vi "Wait For Goal.vi"(6 "Side":T1, 7 "wait time":dbl, 8 "error in":errorcluster, 10 "Goal":dbl[](array[numeric])) -> (0 "error out":errorcluster, 3 "Aborted":bool)   [LabVIEW 2013]
uses:
  ROS/Code/SubVIs/BaxterSide.ctl
  Arm Globals.vi
  ROS/Code/Console/Servers/ServerSubs/(nist) Arm Globals.vi
panel:
  in  "Label":string
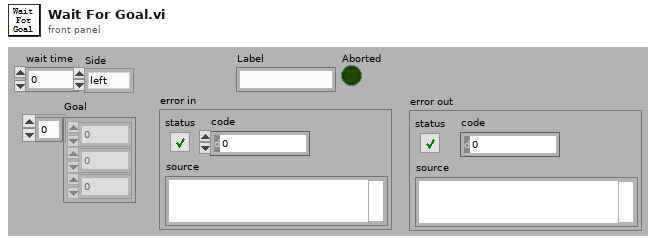
[diagram p1: front panel]
types:
  T1 = typedef "BaxterSide.ctl" = enum16{"left", "right"}
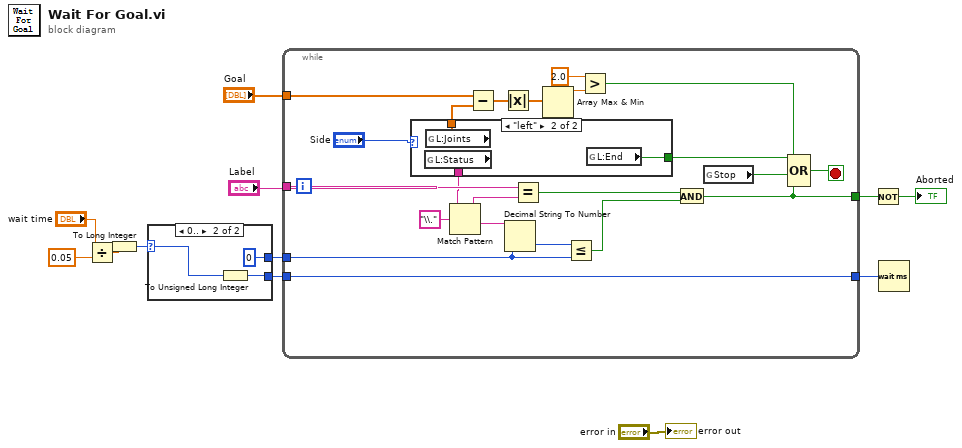
[diagram p0: block diagram]
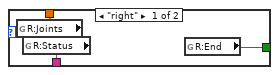
[diagram p2: hidden frame]
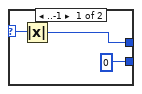
[diagram p3: hidden frame]
diagram:
  n1 = Divide(x="wait time", y=0.05) -> (x/y=w7:dbl)
  n2 = To Long Integer(number=w7) -> (32bit integer=w6:i32)
  n3 = case shown="0.." w6 {
    selector: w6 -> [w15 w17]
    tunnel: [w13 0] -> w11
    tunnel: [u32 0 w18] -> w10
    frame ..-1 {
      n4 = Absolute Value(x=w15) -> (abs(x)=w13:i32)
    }
    frame 0.. {
      n5 = To Unsigned Long Integer(number=w17) -> (unsigned 32bit integer=w18:u32)
    }
  }
  n6 = while {
    tunnel: "Label" -> [w40]
    tunnel: [w28] -> w4
    tunnel: w11 -> [w31]
    tunnel: w10 -> [w30]
    tunnel: [w30] -> w2
    tunnel: "Goal" -> [w24]
    stop <- w38 stop-if-true
    n7 = case shown="\"left\"" "Side" {
      tunnel: [w43 w46] -> w26
      tunnel: [w42 w45] -> w27
      tunnel: [w41 w44] -> w25
      frame "right" {
        n8 = global read "(nist) Arm Globals.vi" "R:Joints"() -> (w41:dbl[])
        n9 = global read "Arm Globals.vi" "R:Status"() -> (w42:string)
        n10 = global read "Arm Globals.vi" "R:End"() -> (w43:bool)
      }
      frame "left" {
        n11 = global read "Arm Globals.vi" "L:Status"() -> (w45:string)
        n12 = global read "(nist) Arm Globals.vi" "L:Joints"() -> (w44:dbl[])
        n13 = global read "Arm Globals.vi" "L:End"() -> (w46:bool)
      }
    }
    n14 = Match Pattern(string=w27, regular expression="\\.") -> (before substring=w36:string, after substring=w35:string)  [unwired: 1 in, 2 out]
    n15 = Subtract(x=w24, y=w25) -> (x-y=w23:dbl[])
    n16 = Absolute Value(x=w23) -> (abs(x)=w22:dbl[])
    n17 = Decimal String To Number(string=w35, default (0L)=w31) -> (number=w34:i32)  [unwired: 1 in, 1 out]
    n18 = Equal?(x=w40, y=w36) -> (x = y?=w33:bool)
    n19 = Array Max & Min(array=w22) -> (max value=w21:dbl)  [unwired: 3 out]
    n20 = Less Or Equal?(x=w34, y=w31) -> (x <= y?=w32:bool)
    n21 = Greater?(x=2.0, y=w21) -> (0:w19:bool)
    n22 = And(x=w33, y=w32) -> (x .and. y?=w28:bool)
    n23 = global read "Arm Globals.vi" "Stop"() -> (w39:bool)
    n24 = Compound Arithmetic op=OR(w19, w26, w39, w28) -> (w38:bool)
  }
  n25 = Not(x=w4) -> (.not. x?=→"Aborted":bool)
  n26 = Wait (ms)(milliseconds to wait=w2) -> ()  [unwired: 1 out]
  "error out" <- "error in"
